vi "DeleteEmptyElement.vi"(8 "error in":errorcluster caption="错误输入", 11 "ArrayIn":string[][](array[string])) -> (0 "error out":errorcluster caption="错误输出", 3 "ArrayOut":string[][](array[string]))   [LabVIEW 2013]
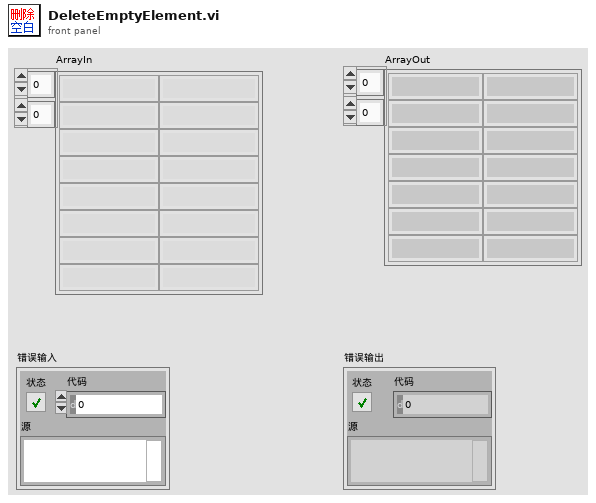
[diagram p1: front panel]
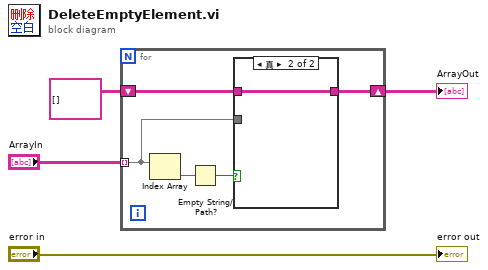
[diagram p0: block diagram]
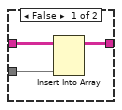
[diagram p2: hidden frame]
diagram:
  n1 = for {
    tunnel: "ArrayIn" -> [w6] mode=indexing
    shift-right: [w5] -> w2
    shift-left: string[][] [] ("ArrayIn") -> [w7]
    n2 = Index Array(array=w6) -> (element=w9:string)  [unwired: 1 in]
    n3 = Empty String/Path?(string/path=w9) -> (empty?=w8:bool)
    n4 = case shown="真" w8 {
      tunnel: w7 -> [w12 w13]
      tunnel: w6 -> [w11 _]
      tunnel: [w10 w13] -> w5
      frame False {
        n5 = Insert Into Array(array=w12, new element=w11) -> (w10:string[][])  [unwired: 2 in]
      }
      frame True {
      }
    }
  }
  "ArrayOut" <- w2
  "error out" <- "error in"
